vi "Initialize.vi"(8 "error in (no error)":errorcluster, 9 "Reset (True)":bool=TRUE, 10 "ID Query (True)":bool=TRUE, 11 "serial number":string) -> (0 "error out":errorcluster, 3 "MC switch refnum out":refnum<k24>)   [LabVIEW 2019, in "Minicircuit RF Switch Box.lvlib"]
doc: "Establishes communication with the instrument and optionally performs an instrument identification query and/or an instrument reset. Several connection can be establish with a switch matrix.\n\n<b>serial number:</b> Optional. The serial number of the USB switch matrix. Can be omitted if only one switch matrix is connected."
uses:
  <instrlib>/LV_Minicircuit_RF_Switch/Minicircuit RF Switch Box.lvlib
  C:/Program Files (x86)/National Instruments/LabVIEW 2019/instr.lib/LV_Minicircuit_RF_Switch/mcl_RF_Switch_Controller_NET45.dll
  mcl_RF_Switch_Controller_NET45.dll
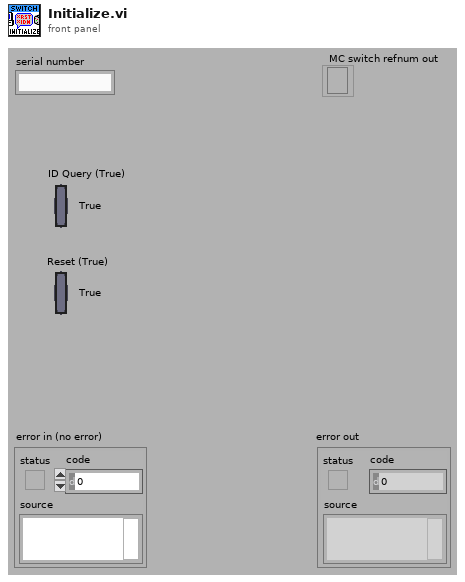
[diagram p1: front panel]
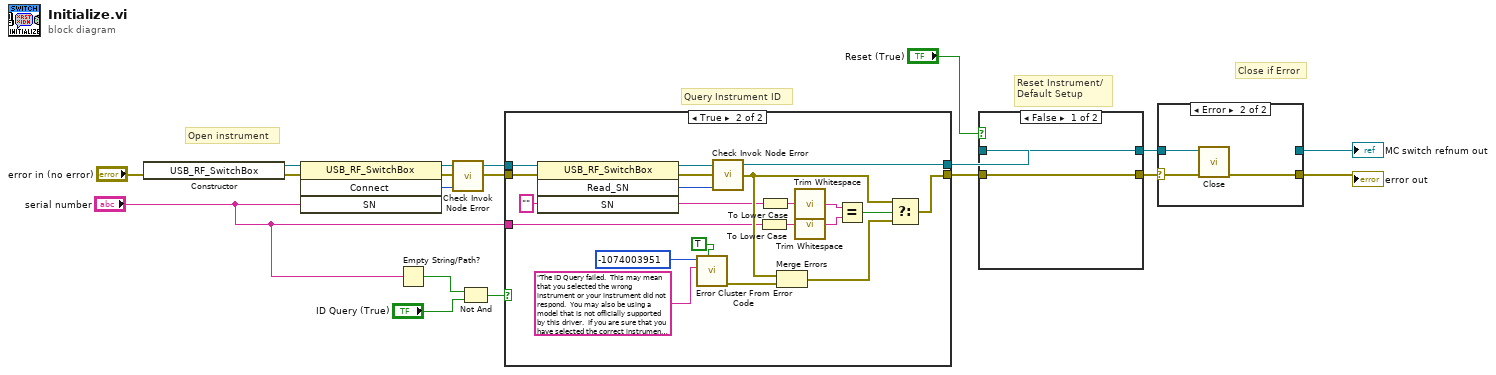
[diagram p0: block diagram]
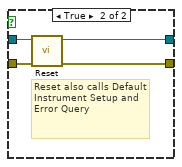
[diagram p4: hidden frame]
diagram:
  # "Close if Error"
  # "Query Instrument ID"
  # "Reset Instrument/\nDefault Setup"
  # "Open instrument"
  n1 = constructor class="USB_RF_SwitchBox"(error in="error in (no error)") -> (reference out=w15:refnum<k24>, error out=w14:errorcluster)  [unwired: 2 in, 1 out]
  n2 = invoke class="USB_RF_SwitchBox" method="Connect"(reference=w15, error in=w14, "SN"="serial number") -> (reference out=w13:refnum<k24>, error out=w11:errorcluster, "Connect"=w9:i32)  [unwired: 1 in, 1 out]
  n3 = Empty String/Path?(string/path="serial number") -> (empty?=w4:bool)
  n4 = call <instrlib>:"Check Invok Node Error.vi"("Connect"=w9, "error in (no error)"=w11, "MC switch refnum in"=w13) -> ("error out"=w10:errorcluster, "MC switch refnum out"=w12:refnum<k24>)  [unwired: 1 in]
  n5 = Not And(1:"ID Query (True)", 2:w4) -> (0:w2:bool)
  n6 = case shown="True" w2 {
    tunnel: w12 -> [w21 w42]
    tunnel: w10 -> [w20 w41]
    tunnel: [w21 w37] -> w7
    tunnel: "serial number" -> [_ w23]
    tunnel: [w20 w27] -> w8
    frame False {
    }
    frame True {
      n7 = invoke class="USB_RF_SwitchBox" method="Read_SN"(reference=w42, error in=w41, "SN"="") -> (reference out=w40:refnum<k24>, error out=w39:errorcluster, "Read_SN"=w38:i32, "SN"=w25:string)  [unwired: 1 in]
      n8 = call <vilib>:"Error Cluster From Error Code.vi"("show call chain? (False)"=TRUE, "error message (\"\")"="The ID Query failed.  This may mean that you selected the wrong instrument or your instrument did not respond.  You may also be using a model that is not officially supported by this driver.  If you are sure that you have selected the correct instrument and it is responding, try disabling the ID Query." ("Source (VI Name)"), "error code (0)"=-1074003951 ("Code")) -> ("error out"=w29:errorcluster)  [unwired: 6 in]
      n9 = call <instrlib>:"Check Invok Node Error.vi"("Connect"=w38, "error in (no error)"=w39, "MC switch refnum in"=w40) -> ("error out"=w30:errorcluster, "MC switch refnum out"=w37:refnum<k24>)  [unwired: 1 in]
      n10 = To Lower Case(string=w23) -> (all lower case string=w24:string)
      n11 = To Lower Case(string=w25) -> (all lower case string=w26:string)
      n12 = Merge Errors(w30, w29) -> (w28:errorcluster)
      n13 = call <vilib>:"Trim Whitespace.vi"("string"=w26) -> ("trimmed string"=w32:string)  [unwired: 1 in]
      n14 = call <vilib>:"Trim Whitespace.vi"("string"=w24) -> ("trimmed string"=w33:string)  [unwired: 1 in]
      n15 = Equal?(x=w32, y=w33) -> (x = y?=w31:bool)
      n16 = Select(t=w30, s=w31, f=w28) -> (s? t:f=w27:errorcluster)
    }
  }
  n17 = case shown="False" "Reset (True)" {
    tunnel: [w44 w48] -> w17
    tunnel: w8 -> [w44 w47]
    tunnel: w7 -> [w43 w46]
    tunnel: [w43 w45] -> w6
    frame False {
    }
    frame True {
      # "Reset also calls Default Instrument Setup and Error Query"
      n18 = call <instrlib>:"Reset.vi"("error in (no error)"=w47, "MC switch refnum in"=w46) -> ("error out"=w48:errorcluster, "MC switch refnum out"=w45:refnum<k24>)  [unwired: 8 in]
    }
  }
  n19 = case shown="Error" w17 {
    selector: w17 -> [w50 w52]
    tunnel: [w50 w53] -> w18
    tunnel: [w49 _] -> w5
    tunnel: w6 -> [w49 w51]
    frame No Error {
    }
    frame Error {
      n20 = call <instrlib>:"Close.vi"("error in (no error)"=w52, "MC switch refnum in"=w51) -> ("error out"=w53:errorcluster)  [unwired: 9 in]
    }
  }
  "error out" <- w18
  "MC switch refnum out" <- w5
